vi "Send Set Mode.vi"(7 "Message Priority (Normal)":T1=enum."Normal", 8 "error in (no error)":errorcluster, 10 "mode":u8(ring) items=["once", "continous"], 11 "Message Enqueuer":refnum<class "Message Enqueuer.lvclass">) -> (0 "error out":errorcluster, 3 "Message Enqueuer out":refnum<class "Message Enqueuer.lvclass">)   [LabVIEW 2015, in "CS++PPG.lvlib" / "Set Mode Msg.lvclass"]
doc: "Sends the <B>CS++PPG.lvlib:Set Mode Msg.lvclass</B> message.\n\n<B>CS++PPG.lvlib:CS++PPG.lvclass:Set Mode.vi</B> Description:\n\nThis Vi sets the mode of the PPG (0 - single run, 1 - continous)."
uses:
  Set Mode Msg.lvclass
  <vilib>/ActorFramework/Message Enqueuer/Message Enqueuer.lvclass
  <vilib>/ActorFramework/Message Enqueuer/Message Priority.ctl
  Set Mode Msg.lvclass/Set Mode Msg.ctl
  <vilib>/ActorFramework/Message Enqueuer/Message Enqueuer.lvclass/Message Enqueuer.ctl
  <vilib>/ActorFramework/Message Priority Queue/Priority Enqueue.vi
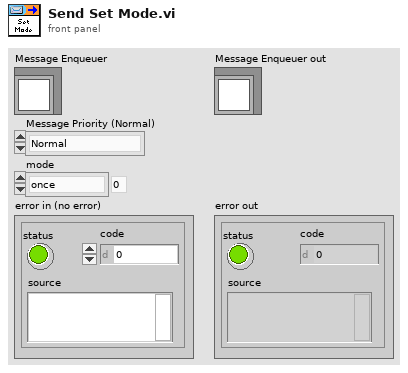
[diagram p1: front panel]
types:
  T1 = typedef "Actor Framework.lvlib/Message Enqueuer.lvclass/Message Priority.ctl" = enum16{"Low", "Normal", "High"}
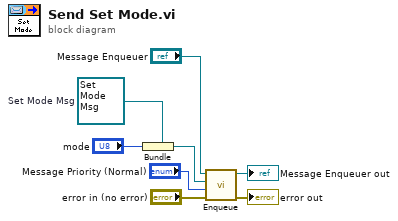
[diagram p0: block diagram]
diagram:
  w2 = refnum<class "Set Mode Msg.lvclass"> refnum  # Set Mode Msg
  n1 = Bundle(cluster=w2, "mode") -> (w5:refnum<class "Set Mode Msg.lvclass">)
  n2 = call <vilib>:"Enqueue.vi"("error in (no error)"="error in (no error)", "Message Priority (Normal)"="Message Priority (Normal)", "Message"=w5, "Message Enqueuer in"="Message Enqueuer") -> ("error out"=→"error out":errorcluster, "Message Enqueuer out"=→"Message Enqueuer out":refnum<class "Message Enqueuer.lvclass">)  [unwired: 6 in]
